vi "Autonomous Independent.vi"() -> ()   [LabVIEW 2014]
doc: "This VI is called when autonomous begins, and will automatically be terminated when autonomous ends. You can carry out timed or sensor driven robot movement independently without needing to return to the caller."
uses:
  <vilib>/Rock Robotics/WPI/SafetyOutput/WPI_SafetyOutputConfigMenu.ctl
  <vilib>/Rock Robotics/WPI/Joystick/WPI_JoystickGetSetRefNum.vi
  <vilib>/Rock Robotics/WPI/RobotDrive/WPI_RobotDriveGetSetRefNum.vi
  <vilib>/Rock Robotics/WPI/Solenoid/Deprecated/WPI_SolenoidSetBool.vi
  <vilib>/Rock Robotics/WPI/RobotDrive/WPI_RobotDriveArcadeDrive_Standard(NoSaturation).vi
panel:
  in  "Value":bool
  out "Current Movement, for debugging":T1 {"Y Joystick Value" scale=1.0..-1.0; "X Joystick Value" scale=-1.0..1.0}
  in  "Array of robot movements":T2(array[cluster]) {"Y Joystick Value" scale=1.0..-1.0; "X Joystick Value" scale=-1.0..1.0}
  # "Be sure to right-click and choose Data Operations>>Make Current Value default if you want to save the array values with the VI"
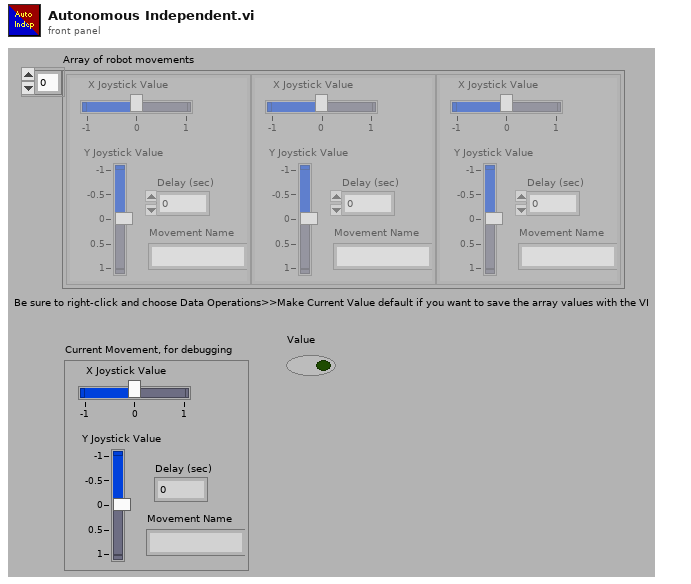
[diagram p1: front panel]
types:
  T1 = cluster{"X Joystick Value":dbl, "Y Joystick Value":dbl, "Delay (sec)":dbl, "Movement Name":string}
  T2 = cluster{"X Joystick Value":dbl, "Y Joystick Value":dbl, "Delay (sec)":dbl, "Movement Name":string}[]
  T3 = typedef "WPI_SafetyOutputConfigMenu.ctl" = enum16{"Enable", "Disable"}
  T4 = typedef "WPI_MotorControlDeviceRef.ctl" = cluster{"DeviceStatus":errorcluster, "Type":T5, "PWM":cluster{"Controller":T6, "PWM Channel":T7, "DeadBand":T8}, "CAN":cluster{"Device Number":u8, "Control Mode":T9, "Semaphore":T10, "Max Vout":dbl, "TalonSRX Control Mode":T11}, "Invert":bool, "TransformRef":T12, "InvTransformRef":T12}
  T5 = typedef "WPI_MotorControlType.ctl" = enum16{"PWM", "CAN", "CANTalonSRX"}
  T6 = typedef "FPGA_TypedefDigitalModule.ctl" = enum16{"Controller 1"}
  T7 = typedef "FPGA_DIOPWMChannel.ctl" = enum8{"PWM 0", "PWM 1", "PWM 2", "PWM 3", "PWM 4", "PWM 5", "PWM 6", "PWM 7", "PWM 8", "PWM 9", "PWM MXP 0", "PWM MXP 1", "PWM MXP 2", "PWM MXP 3", "PWM MXP 4", "PWM MXP 5", "PWM MXP 6", "PWM MXP 7", "PWM MXP 8", "PWM MXP 9", "Invalid"}
  T8 = typedef "WPI_PWMDeadband.ctl" = cluster{"Name":string, "maxPositivePwm":i32, "minPositivePwm":i32, "centerPwm":i32, "maxNegativePwm":i32, "minNegativePwm":i32, "angularRange":u16}
  T9 = typedef "WPI_CANJaguar_ControlMode.ctl" = enum8{"Percent VBus", "Current", "Speed", "Position", "Voltage"}
  T10 = typedef "Semaphore RefNum" = refnum<k1>
  T11 = typedef "WPI_CANTalonSRX_APIControlMode.ctl" = enum8{"Percent VBus", "Speed", "Position", "Slave", "Unchanged / Invalid"}
  T12 = typedef "WPI_PWMTransform_ConPane.ctl" = refnum<vi>
  T13 = typedef "WPI_SolenoidDevRef.ctl" = cluster{"DevStatus":errorcluster, "Pneumatics Control Module":u8, "Forward Solenoid Channel":T14, "Reverse Solenoid Channel":T14}
  T14 = typedef "WPI_SolenoidChannel.ctl" = enum8{"Solenoid 0", "Solenoid 1", "Solenoid 2", "Solenoid 3", "Solenoid 4", "Solenoid 5", "Solenoid 6", "Solenoid 7", "Invalid"}
  T15 = typedef "WPI_RobotDriveDevRef.ctl" = cluster{"DevStatus":errorcluster, "Motors[]":T4[], "Square Inputs":bool, "Max Output":dbl}
  T16 = typedef "WPI_JoystickDevRef.ctl" = cluster{"Device":T17}
  T17 = typedef "WPI_JoystickDeviceEnum.ctl" = enum16{"USB 0", "USB 1", "USB 2", "USB 3", "USB 4", "USB 5"}
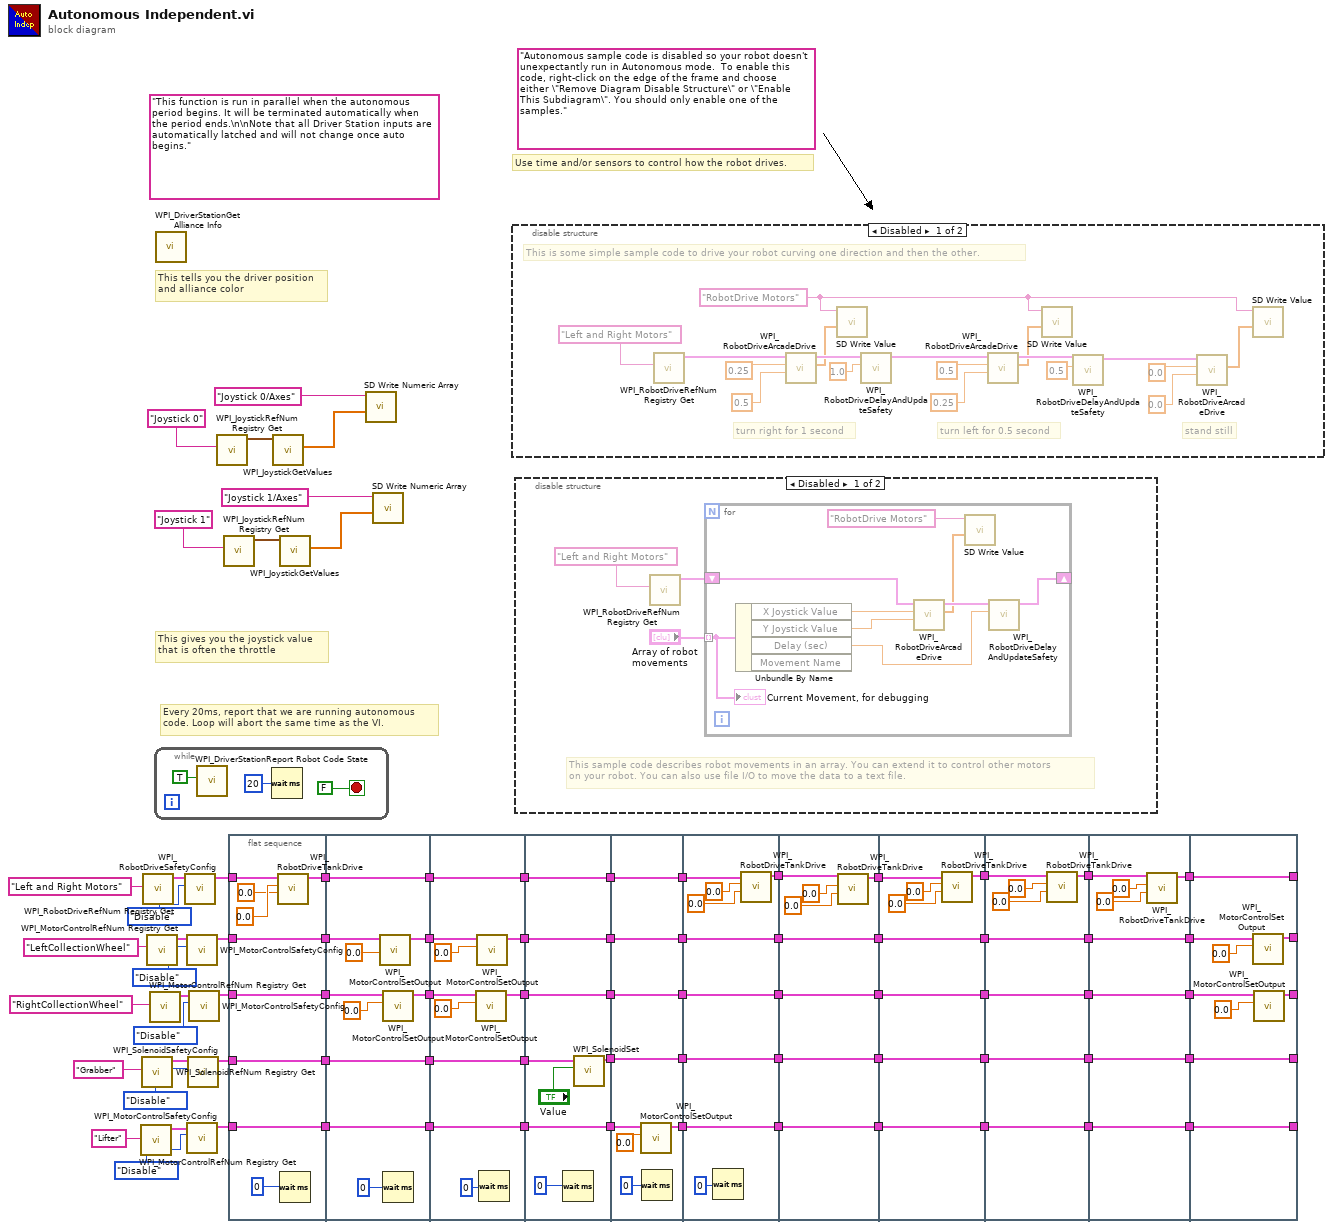
[diagram p0: block diagram]
diagram:
  (unwired) "Autonomous sample code is disabled so your robot doesn't unexpectantly run in Autonomous mode.  To enable this code, right-click on the edge of the frame and choose either \"Remove Diagram Disable Structure\" or \"Enable This Subdiagram\". You should only enable one of the samples."
  (unwired) "This function is run in parallel when the autonomous period begins. It will be terminated automatically when the period ends.\n\nNote that all Driver Station inputs are automatically latched and will not change once auto begins."
  # "Every 20ms, report that we are running autonomous\ncode. Loop will abort the same time as the VI."
  # "This gives you the joystick value\nthat is often the throttle"
  # "Use time and/or sensors to control how the robot drives."
  # "This tells you the driver position\nand alliance color"
  n1 = call <vilib>:"WPI_MotorControlRefNum Registry Get.vi"("refnum name"="Lifter") -> ("MotorControlDevRef"=w42:T4)  [unwired: 9 in, 1 out]
  n2 = call <vilib>:"WPI_SolenoidRefNum Registry Get.vi"("refnum name"="Grabber") -> ("SolenoidDevRef"=w49:T13)  [unwired: 9 in, 1 out]
  n3 = call <vilib>:"WPI_RobotDriveRefNum Registry Get.vi"("refnum name"="Left and Right Motors") -> ("RobotDriveDevRef"=w70:T15)  [unwired: 9 in, 1 out]
  n4 = call <vilib>:"WPI_MotorControlRefNum Registry Get.vi"("refnum name"="LeftCollectionWheel") -> ("MotorControlDevRef"=w65:T4)  [unwired: 9 in, 1 out]
  n5 = call <vilib>:"WPI_MotorControlRefNum Registry Get.vi"("refnum name"="RightCollectionWheel") -> ("MotorControlDevRef"=w59:T4)  [unwired: 9 in, 1 out]
  n6 = while {
    stop <- FALSE stop-if-true
    n7 = call <vilib>:"WPI_DriverStationReport Robot Code State.vi"("Autonomous"=TRUE) -> ()  [unwired: 10 in, 1 out]
    n8 = Wait (ms)(milliseconds to wait=u32 20) -> ()  [unwired: 1 out]
  }
  n9 = call <vilib>:"WPI_DriverStationGet Alliance Info.vi"() -> ()  [unwired: 12 out]
  n10 = call <vilib>:"WPI_RobotDriveSafetyConfig.vi"("mode"=WPI_SafetyOutputConfigMenu."Disable", "RobotDriveDevRef"=w70) -> ("RobotDriveDevRef"=w69:T15)  [unwired: 8 in, 1 out]
  n11 = call <vilib>:"WPI_MotorControlSafetyConfig.vi"("mode"=WPI_SafetyOutputConfigMenu."Disable", "MotorControlDevRef"=w65) -> ("MotorControlDevRef"=w63:T4)  [unwired: 8 in, 1 out]
  n12 = call <vilib>:"WPI_MotorControlSafetyConfig.vi"("mode"=WPI_SafetyOutputConfigMenu."Disable", "MotorControlDevRef"=w42) -> ("MotorControlDevRef"=w39:T4)  [unwired: 8 in, 1 out]
  n13 = call <vilib>:"WPI_SolenoidSafetyConfig.vi"("mode"=WPI_SafetyOutputConfigMenu."Disable", "SolenoidDevRef"=w49) -> ("SolenoidDevRef 2"=w48:T13)  [unwired: 8 in, 1 out]
  n14 = call <vilib>:"WPI_MotorControlSafetyConfig.vi"("mode"=WPI_SafetyOutputConfigMenu."Disable", "MotorControlDevRef"=w59) -> ("MotorControlDevRef"=w58:T4)  [unwired: 8 in, 1 out]
  n15 = call <vilib>:"WPI_JoystickRefNum Registry Get.vi"("refnum name"="Joystick 0") -> ("JoystickDevRef"=w77:T16)  [unwired: 1 in, 9 out]
  n16 = call <vilib>:"WPI_JoystickRefNum Registry Get.vi"("refnum name"="Joystick 1") -> ("JoystickDevRef"=w73:T16)  [unwired: 1 in, 9 out]
  n17 = flat-sequence {
    tunnel: w69 -> [w90]
    tunnel: [w87] -> w66
    tunnel: w63 -> [w86]
    tunnel: [w86] -> w61
    tunnel: w58 -> [w85]
    tunnel: [w85] -> w57
    tunnel: w48 -> [w84]
    tunnel: [w84] -> w45
    tunnel: w39 -> [w83]
    tunnel: [w83] -> w38
    tunnel: w66 -> [w100]
    tunnel: w61 -> [w99]
    tunnel: w57 -> [w96]
    tunnel: [w100] -> w55
    tunnel: [w97] -> w54
    tunnel: [w95] -> w53
    tunnel: w45 -> [w93]
    tunnel: [w93] -> w44
    tunnel: w38 -> [w92]
    tunnel: [w92] -> w37
    tunnel: w55 -> [w110]
    tunnel: w54 -> [w108]
    tunnel: w53 -> [w109]
    tunnel: [w110] -> w52
    tunnel: [w105] -> w51
    tunnel: [w104] -> w50
    tunnel: w44 -> [w103]
    tunnel: [w103] -> w43
    tunnel: w37 -> [w102]
    tunnel: [w102] -> w36
    tunnel: w52 -> [w118]
    tunnel: w51 -> [w117]
    tunnel: w50 -> [w116]
    tunnel: w43 -> [w115]
    tunnel: w36 -> [w112]
    tunnel: [w118] -> w35
    tunnel: [w117] -> w34
    tunnel: [w116] -> w33
    tunnel: [w114] -> w32
    tunnel: [w112] -> w31
    tunnel: w35 -> [w126]
    tunnel: w34 -> [w125]
    tunnel: w33 -> [w124]
    tunnel: w32 -> [w123]
    tunnel: w31 -> [w122]
    tunnel: [w126] -> w30
    tunnel: [w125] -> w29
    tunnel: [w124] -> w28
    tunnel: [w123] -> w27
    tunnel: [w121] -> w26
    tunnel: w30 -> [w131]
    tunnel: w29 -> [w135]
    tunnel: w28 -> [w134]
    tunnel: w27 -> [w133]
    tunnel: w26 -> [w132]
    tunnel: [w135] -> w25
    tunnel: [w134] -> w24
    tunnel: [w133] -> w23
    tunnel: [w132] -> w22
    tunnel: [w130] -> w21
    tunnel: w25 -> [w143]
    tunnel: w24 -> [w142]
    tunnel: w23 -> [w141]
    tunnel: w22 -> [w140]
    tunnel: w21 -> [w137]
    tunnel: [w143] -> w20
    tunnel: [w142] -> w19
    tunnel: [w141] -> w18
    tunnel: [w140] -> w17
    tunnel: [w136] -> w16
    tunnel: w20 -> [w151]
    tunnel: w19 -> [w150]
    tunnel: w18 -> [w149]
    tunnel: w17 -> [w148]
    tunnel: w16 -> [w145]
    tunnel: [w151] -> w15
    tunnel: [w150] -> w14
    tunnel: [w149] -> w13
    tunnel: [w148] -> w12
    tunnel: [w144] -> w11
    tunnel: w15 -> [w159]
    tunnel: w14 -> [w158]
    tunnel: w13 -> [w157]
    tunnel: w12 -> [w156]
    tunnel: w11 -> [w155]
    tunnel: [w159] -> w10
    tunnel: [w158] -> w9
    tunnel: [w157] -> w8
    tunnel: [w156] -> w7
    tunnel: [w154] -> w6
    tunnel: w10 -> [w167]
    tunnel: w9 -> [w166]
    tunnel: w8 -> [w165]
    tunnel: w7 -> [w164]
    tunnel: w6 -> [w163]
    tunnel: [w167] -> w5
    tunnel: [w166] -> w4
    tunnel: [w165] -> w3
    tunnel: [w164] -> w2
    tunnel: [w162] -> w1
    tunnel: [w174] -> _
    tunnel: [w175] -> _
    tunnel: [w176] -> _
    tunnel: w5 -> [w173]
    tunnel: w4 -> [w171]
    tunnel: w3 -> [w176]
    tunnel: w2 -> [w175]
    tunnel: w1 -> [w174]
    tunnel: [w172] -> _
    tunnel: [w170] -> _
    frame #0 {
      n18 = call <vilib>:"WPI_RobotDriveTankDrive.vi"("Right axis value"=0.0, "Left axis value"=0.0, "RobotDriveDevRef"=w90) -> ("RobotDriveDevRef"=w87:T15)  [unwired: 6 in, 2 out]
      n19 = Wait (ms)(milliseconds to wait=0) -> ()  [unwired: 1 out]
    }
    frame #1 {
      n20 = call <vilib>:"WPI_MotorControlSetOutput.vi"("Output"=0.0, "MotorControlDevRef"=w99) -> ("MotorControlDevRef"=w97:T4)  [unwired: 7 in, 2 out]
      n21 = call <vilib>:"WPI_MotorControlSetOutput.vi"("Output"=0.0, "MotorControlDevRef"=w96) -> ("MotorControlDevRef"=w95:T4)  [unwired: 7 in, 2 out]
      n22 = Wait (ms)(milliseconds to wait=0) -> ()  [unwired: 1 out]
    }
    frame #2 {
      n23 = call <vilib>:"WPI_MotorControlSetOutput.vi"("Output"=0.0, "MotorControlDevRef"=w109) -> ("MotorControlDevRef"=w104:T4)  [unwired: 7 in, 2 out]
      n24 = call <vilib>:"WPI_MotorControlSetOutput.vi"("Output"=0.0, "MotorControlDevRef"=w108) -> ("MotorControlDevRef"=w105:T4)  [unwired: 7 in, 2 out]
      n25 = Wait (ms)(milliseconds to wait=0) -> ()  [unwired: 1 out]
    }
    frame #3 {
      n26 = Wait (ms)(milliseconds to wait=0) -> ()  [unwired: 1 out]
      n27 = call-poly <vilib>:"WPI_SolenoidSet.vi"("Value"="Value", "SolenoidDevRef"=w115) -> ("SolenoidDevRef"=w114:T13)  [unwired: 8 in, 1 out]
    }
    frame #4 {
      n28 = call <vilib>:"WPI_MotorControlSetOutput.vi"("Output"=0.0, "MotorControlDevRef"=w122) -> ("MotorControlDevRef"=w121:T4)  [unwired: 7 in, 2 out]
      n29 = Wait (ms)(milliseconds to wait=0) -> ()  [unwired: 1 out]
    }
    frame #5 {
      n30 = Wait (ms)(milliseconds to wait=0) -> ()  [unwired: 1 out]
      n31 = call <vilib>:"WPI_RobotDriveTankDrive.vi"("Right axis value"=0.0, "Left axis value"=0.0, "RobotDriveDevRef"=w131) -> ("RobotDriveDevRef"=w130:T15)  [unwired: 6 in, 2 out]
    }
    frame #6 {
      n32 = call <vilib>:"WPI_RobotDriveTankDrive.vi"("Right axis value"=0.0, "Left axis value"=0.0, "RobotDriveDevRef"=w137) -> ("RobotDriveDevRef"=w136:T15)  [unwired: 6 in, 2 out]
    }
    frame #7 {
      n33 = call <vilib>:"WPI_RobotDriveTankDrive.vi"("Right axis value"=0.0, "Left axis value"=0.0, "RobotDriveDevRef"=w145) -> ("RobotDriveDevRef"=w144:T15)  [unwired: 6 in, 2 out]
    }
    frame #8 {
      n34 = call <vilib>:"WPI_RobotDriveTankDrive.vi"("Right axis value"=0.0, "Left axis value"=0.0, "RobotDriveDevRef"=w155) -> ("RobotDriveDevRef"=w154:T15)  [unwired: 6 in, 2 out]
    }
    frame #9 {
      n35 = call <vilib>:"WPI_RobotDriveTankDrive.vi"("Right axis value"=0.0, "Left axis value"=0.0, "RobotDriveDevRef"=w163) -> ("RobotDriveDevRef"=w162:T15)  [unwired: 6 in, 2 out]
    }
    frame #10 {
      n36 = call <vilib>:"WPI_MotorControlSetOutput.vi"("Output"=0.0, "MotorControlDevRef"=w173) -> ("MotorControlDevRef"=w172:T4)  [unwired: 7 in, 2 out]
      n37 = call <vilib>:"WPI_MotorControlSetOutput.vi"("Output"=0.0, "MotorControlDevRef"=w171) -> ("MotorControlDevRef"=w170:T4)  [unwired: 7 in, 2 out]
    }
  }
  n38 = call <vilib>:"WPI_JoystickGetValues.vi"("JoystickDevRef"=w77) -> ("Axes"=w75:dbl[])  [unwired: 6 in, 4 out]
  n39 = call <vilib>:"WPI_JoystickGetValues.vi"("JoystickDevRef"=w73) -> ("Axes"=w71:dbl[])  [unwired: 6 in, 4 out]
  n40 = call <vilib>:"SD Write Numeric Array.vi"("Numeric Array"=w75, "Name"="Joystick 0/Axes") -> ()  [unwired: 8 in, 2 out]
  n41 = call <vilib>:"SD Write Numeric Array.vi"("Numeric Array"=w71, "Name"="Joystick 1/Axes") -> ()  [unwired: 8 in, 2 out]
  n42 = disable-structure shown="Disabled" {
    frame Disabled {
      w180 = "RobotDrive Motors" ("Name")
      # "This is some simple sample code to drive your robot curving one direction and then the other."
      # "stand still"
      # "turn left for 0.5 second"
      # "turn right for 1 second"
      n43 = call <vilib>:"WPI_RobotDriveRefNum Registry Get.vi"("refnum name"="Left and Right Motors") -> ("RobotDriveDevRef"=w181:T15)  [unwired: 1 in, 9 out]
      n44 = call-poly <vilib>:"WPI_RobotDriveArcadeDrive.vi"("Y axis value"=0.5 ("X axis value"), "X axis value"=0.25, "RobotDriveDevRef"=w181) -> ("Motor Values"=w179:dbl[], "RobotDriveDevRef"=w188:T15)  [unwired: 1 in, 6 out]
      n45 = call-poly <vilib>:"SD Write Value.vi"("Numeric Array"=w179, "Name"=w180) -> ()  [unwired: 8 in, 2 out]
      n46 = call <vilib>:"WPI_RobotDriveDelayAndUpdateSafety.vi"("Delay (s)"=1.0, "RobotDriveDevRef"=w188) -> ("RobotDriveDevRef 2"=w187:T15)  [unwired: 8 in, 1 out]
      n47 = call-poly <vilib>:"WPI_RobotDriveArcadeDrive.vi"("Y axis value"=0.25 ("X axis value"), "X axis value"=0.5, "RobotDriveDevRef"=w187) -> ("Motor Values"=w178:dbl[], "RobotDriveDevRef"=w186:T15)  [unwired: 1 in, 6 out]
      n48 = call-poly <vilib>:"SD Write Value.vi"("Numeric Array"=w178, "Name"=w180) -> ()  [unwired: 8 in, 2 out]
      n49 = call <vilib>:"WPI_RobotDriveDelayAndUpdateSafety.vi"("Delay (s)"=0.5, "RobotDriveDevRef"=w186) -> ("RobotDriveDevRef 2"=w185:T15)  [unwired: 8 in, 1 out]
      n50 = call-poly <vilib>:"WPI_RobotDriveArcadeDrive.vi"("Y axis value"=0.0 ("X axis value"), "X axis value"=0.0, "RobotDriveDevRef"=w185) -> ("Motor Values"=w177:dbl[])  [unwired: 1 in, 7 out]
      n51 = call-poly <vilib>:"SD Write Value.vi"("Numeric Array"=w177, "Name"=w180) -> ()  [unwired: 8 in, 2 out]
    }
    frame Enabled {
    }
  }
  n52 = disable-structure shown="Disabled" {
    frame Disabled {
      # "This sample code describes robot movements in an array. You can extend it to control other motors\non your robot. You can also use file I/O to move the data to a text file."
      n53 = call <vilib>:"WPI_RobotDriveRefNum Registry Get.vi"("refnum name"="Left and Right Motors") -> ("RobotDriveDevRef"=w196:T15)  [unwired: 1 in, 9 out]
      n54 = for {
        shift-right: [w203] -> _
        shift-left: w196 -> [w204]
        tunnel: "Array of robot movements" -> [w199] mode=indexing
        n55 = Unbundle By Name(w199) -> ("X Joystick Value"=w202:dbl, "Y Joystick Value"=w201:dbl, "Delay (sec)"=w200:dbl)  [unwired: 1 out]
        n56 = call-poly <vilib>:"WPI_RobotDriveArcadeDrive.vi"("Y axis value"=w201, "X axis value"=w202, "RobotDriveDevRef"=w204) -> ("Motor Values"=w198:dbl[], "RobotDriveDevRef"=w205:T15)  [unwired: 1 in, 6 out]
        n57 = call-poly <vilib>:"SD Write Value.vi"("Numeric Array"=w198, "Name"="RobotDrive Motors") -> ()  [unwired: 8 in, 2 out]
        n58 = call <vilib>:"WPI_RobotDriveDelayAndUpdateSafety.vi"("Delay (s)"=w200, "RobotDriveDevRef"=w205) -> ("RobotDriveDevRef 2"=w203:T15)  [unwired: 8 in, 1 out]
        "Current Movement, for debugging" <- w199
      }
    }
    frame Enabled {
    }
  }
